vi "Configure.vi"(8 "error in (no error)":errorcluster, 11 "Measurement in":refnum<class "Measurement.lvclass">) -> (0 "error out":errorcluster, 3 "Measurement out":refnum<class "Measurement.lvclass">)   [LabVIEW 2026, in "Measurement Actor.lvlib" / "Measurement.lvclass"]
doc: "Override configure.vi to setup any parameters for a measurement before acquiring.\n\nConfigure.vi is called by the 'Initialize Measurement Actor Core.vi,' which executes before Actor Core of the root measurement class. The root configure method populates the basic Measurement UI with information such as the hardware device in use and the name of the measurement. The base configure method calls 'Acquire.vi' once execution is complete. If beginning a recurring acquisition, it reset the iteration count to zero."
uses:
  Measurement.lvclass
  Measurement.lvclass/Measurement.ctl
  Messages/Acquire Msg/Acquire Msg.lvclass
  Hardware/Hardware.lvclass
  <vilib>/ActorFramework/Actor/Actor.lvclass
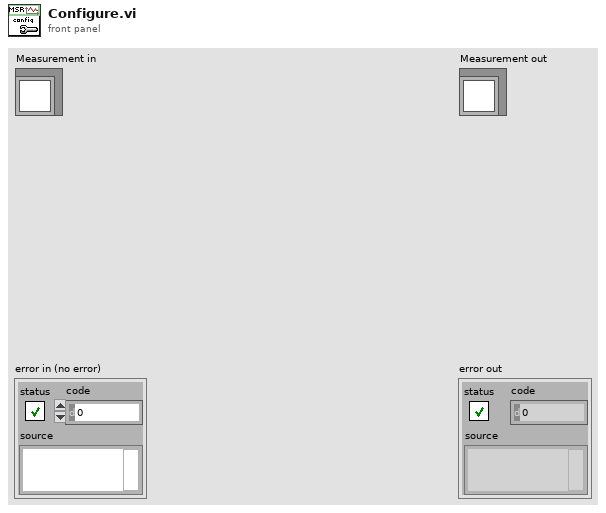
[diagram p1: front panel]
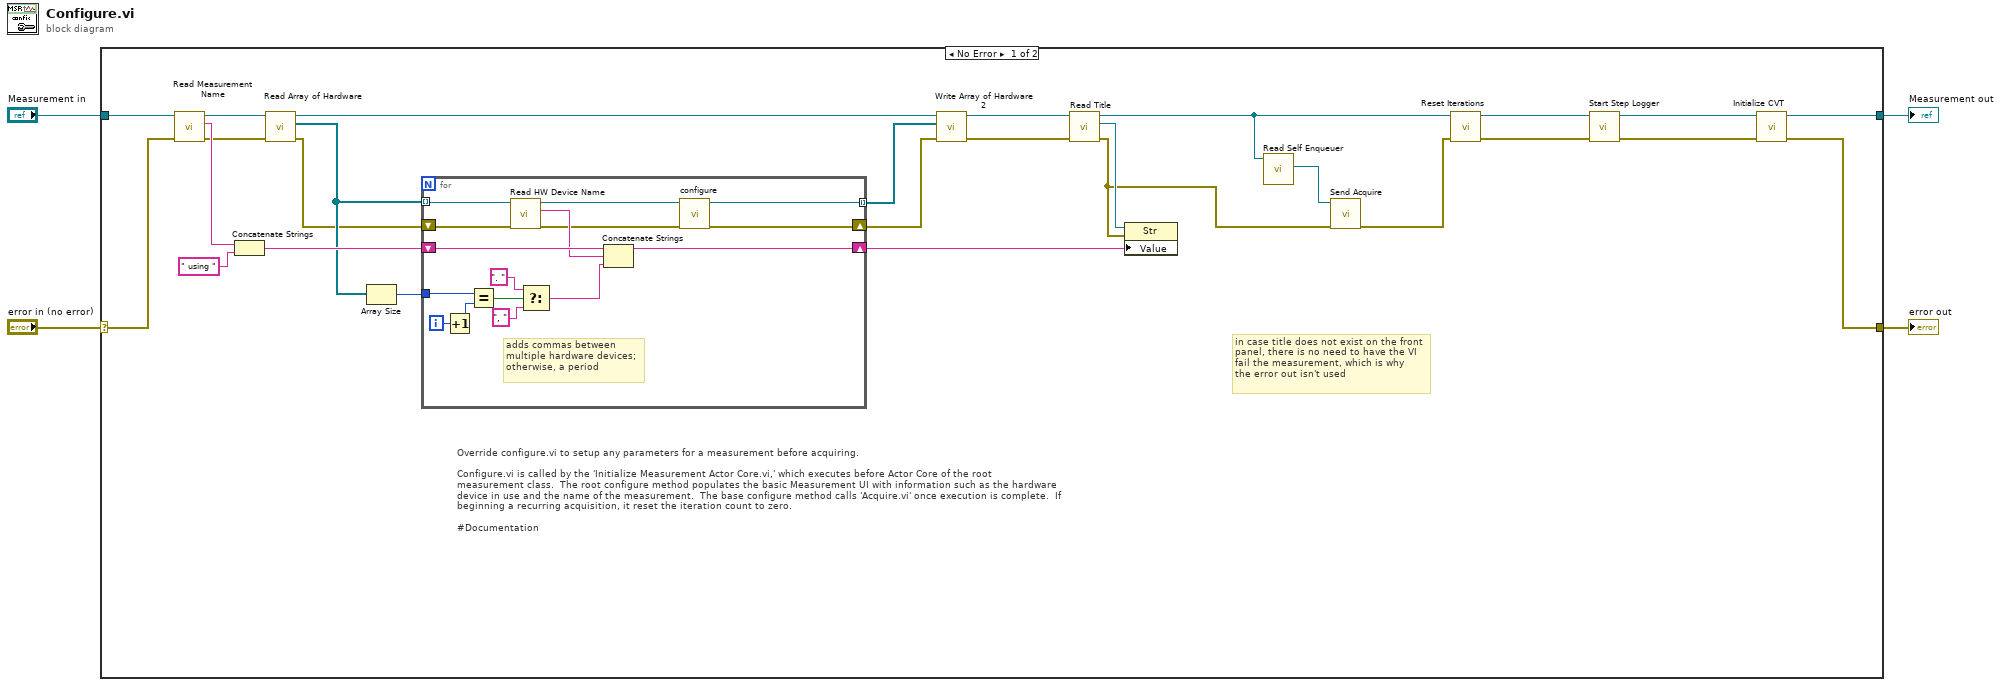
[diagram p0: block diagram]
diagram:
  n1 = case shown="No Error" "error in (no error)" {
    selector: "error in (no error)" -> [w20 w48]
    tunnel: [w12 w48] -> w3
    tunnel: [w10 w47] -> w1
    tunnel: "Measurement in" -> [w29 w47]
    frame No Error {
      # "Override configure.vi to setup any parameters for a measurement before acquiring.\n\nConfigure.vi is called by the 'Initialize Measurement Actor Core.vi,' which executes before Actor Core of the root measurement class.  The root configure method populates the basic Measurement UI with information such as the hardware device in use and the name of the measurement.  The base configure method calls 'Acquire.vi' once execution is complete.  If beginning a recurring acquisition, it reset the iteration count to zero.\n\n#Documentation"
      # "in case title does not exist on the front\npanel, there is no need to have the VI\nfail the measurement, which is why\nthe error out isn't used"
      n2 = call "Read Measurement Name.vi"("error in (no error)"=w20, "Measurement in"=w29) -> ("error out"=w21:errorcluster, "Measurement Name"=w24:string, "Measurement out"=w28:refnum<class "Measurement.lvclass">)  [unwired: 7 in]
      n3 = Concatenate Strings(w24, " using " ("string")) -> (w23:string)
      n4 = call "Read Array of Hardware.vi"("error in (no error)"=w21, "Measurement in"=w28) -> ("error out"=w6:errorcluster, "Array of Hardware"=w18:refnum<class "Hardware.lvclass">[], "Measurement out"=w27:refnum<class "Measurement.lvclass">)  [unwired: 7 in]
      n5 = Array Size(array=w18) -> (size(s)=w17:i32)
      n6 = for {
        tunnel: w18 -> [w46] mode=indexing
        shift-right: [w45] -> w26
        shift-left: w23 -> [w44]
        tunnel: w17 -> [w40]
        tunnel: [w34] -> w7 mode=indexing
        shift-right: [w31] -> w5
        shift-left: w6 -> [w33]
        i -> [w42]
        # "adds commas between\nmultiple hardware devices;\notherwise, a period"
        n7 = Increment(x=w42) -> (x+1=w41:i32)
        n8 = Equal?(x=w40, y=w41) -> (x = y?=w39:bool)
        n9 = call "Read HW Device Name.vi"("error in (no error)"=w33, "Analog in"=w46) -> ("error out"=w32:errorcluster, "Device Name"=w43:string, "Analog out"=w35:refnum<class "Hardware.lvclass">)  [unwired: 7 in]
        n10 = Select(t=". " ("string"), s=w39, f=", " ("string")) -> (s? t:f=w38:string)
        n11 = Concatenate Strings(w44, w43, w38) -> (w45:string)
        n12 = call-dynamic "configure.vi"("error in (no error)"=w32, "Hardware in"=w35) -> ("error out"=w31:errorcluster, "Hardware out"=w34:refnum<class "Hardware.lvclass">)  [unwired: 8 in]
      }
      n13 = call "Write Array of Hardware 2.vi"("Array of Hardware"=w7, "Measurement in"=w27) -> ("Measurement out"=w8:refnum<class "Measurement.lvclass">)  [unwired: 8 in, 1 out]
      n14 = call "Read Title.vi"("error in (no error)"=w5, "Measurement in"=w8) -> ("error out"=w16:errorcluster, "Title"=w30:refnum<vi>, "Measurement out"=w19:refnum<class "Measurement.lvclass">)  [unwired: 7 in]
      n15 = property class="Str"(reference=w30, error in=w16, "Value"=w26) -> ()  [unwired: 2 out]
      n16 = call <vilib>:"Read Self Enqueuer.vi"("Actor"=w19) -> ("Self Enqueuer"=w22:refnum<class "Message Enqueuer.lvclass">)  [unwired: 10 in]
      n17 = call "Send Acquire.vi"("error in (no error)"=w16, "Message Enqueuer in"=w22) -> ("error out"=w15:errorcluster)  [unwired: 8 in, 1 out]
      n18 = call "Reset Iterations.vi"("error in (no error)"=w15, "Measurement in"=w19) -> ("error out"=w14:errorcluster, "Measurement out"=w11:refnum<class "Measurement.lvclass">)  [unwired: 8 in]
      n19 = call "Start Step Logger.vi"("error in (no error)"=w14, "Measurement in"=w11) -> ("error out"=w13:errorcluster, "Measurement out"=w9:refnum<class "Measurement.lvclass">)  [unwired: 8 in]
      n20 = call "Initialize CVT.vi"("error in (no error)"=w13, "Measurement in"=w9) -> ("error out"=w12:errorcluster, "Measurement out"=w10:refnum<class "Measurement.lvclass">)  [unwired: 8 in]
    }
    frame Error {
    }
  }
  "error out" <- w3
  "Measurement out" <- w1
